vi "RegisterEvent_test.vi"() -> ()   [LabVIEW 2018]
panel:
  out "Picture":picture
  out "Numeric":i32
  in  "stop":bool
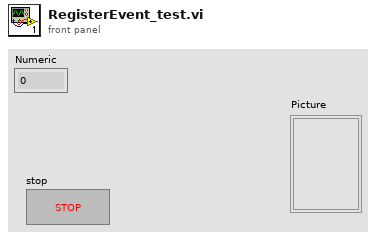
[diagram p1: front panel]
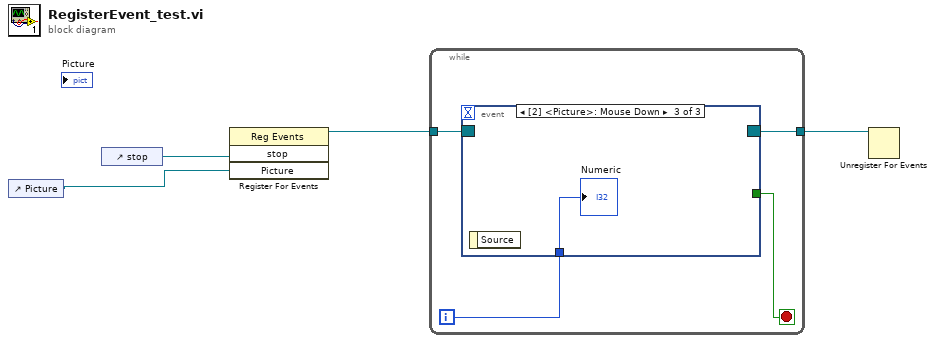
[diagram p0: block diagram]
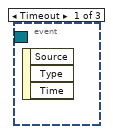
[diagram p2: hidden frame]
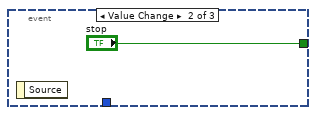
[diagram p3: hidden frame]
diagram:
  n1 = control-ref of="Picture"() -> (w2:refnum<vi>)
  n2 = control-ref of="stop"() -> (w3:refnum<vi>)
  n3 = register-events(w3, w2) -> (reference out=w4:refnum<event-registration>)  [unwired: 2 in, 1 out]
  n4 = while {
    tunnel: w4 -> [w7]
    tunnel: [w5] -> w1
    i -> [w6]
    stop <- w8 stop-if-true
    n5 = event shown="[2] <Picture>: Mouse Down" {
      selector: w7 -> [_ _ _]
      dyn-events: [_ _ _] -> w5
      timeout: _ -> [_ _ _]
      tunnel: [_ "stop" _] -> w8
      tunnel: w6 -> [_ _ w10]
      event Timeout {
        n6 = event-data() -> ()  [unwired: 1 in, 3 out]
      }
      event Value Change {
        n7 = event-data() -> ()  [unwired: 1 in, 1 out]
      }
      event Mouse Down {
        n8 = event-data() -> ()  [unwired: 1 in, 1 out]
        "Numeric" <- w10
      }
    }
  }
  n9 = Unregister For Events(event registration refnum=w1) -> ()  [unwired: 1 in, 1 out]
